vi "niRFUtil WFM Average (DVR) (complex).vi"(0 "Avg State Element DVR":T1, 5 "Data In":T2 format="%.2f", 7 "Average Mode":enum16{"Exponential", "Repeat"}(ring), 11 "error in (no error)":errorcluster, 12 "Reset?":bool=TRUE, 13 "Initialize?":bool=TRUE) -> (6 "Average Data Out":T2 format="%.2f", 8 "Average Count":i32, 15 "error out":errorcluster)   [LabVIEW 2015, in "niRFUtil.lvlib"]
doc: "(c) Copyright 2006, National Instruments, Inc. This VI may not be duplicated, sold, or distributed without written consent from National Instruments."
uses:
  niRFUtil.lvlib
  Includes/niRFUtil INC Complex Array.ctl
  Includes/niRFUtil INC Average State Reference (complex).ctl
  Includes/niRFUtil INC Average State Data (complex).ctl
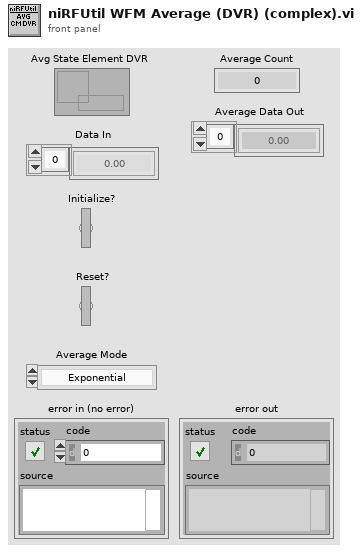
[diagram p1: front panel]
types:
  T1 = typedef "niRFUtil.lvlib/niRFUtil INC Average State Reference (complex).ctl" = refnum<data-value>
  T2 = typedef "niRFUtil.lvlib/niRFUtil INC Complex Array.ctl" = csg[]
  T3 = typedef "niRFUtil.lvlib/niRFUtil INC Average State Data (complex).ctl" = cluster{"Accumulator":T2, "Count":i32}
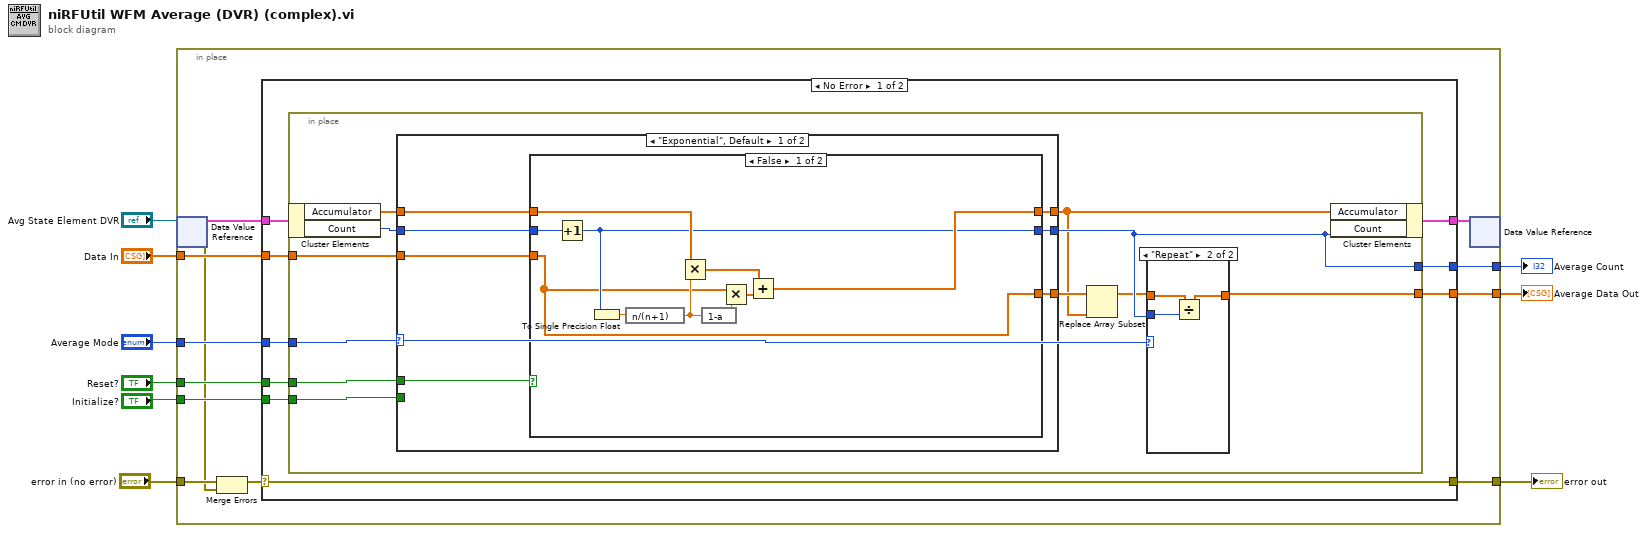
[diagram p0: block diagram]
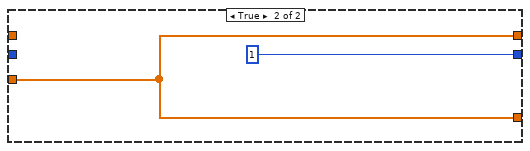
[diagram p2: hidden frame]
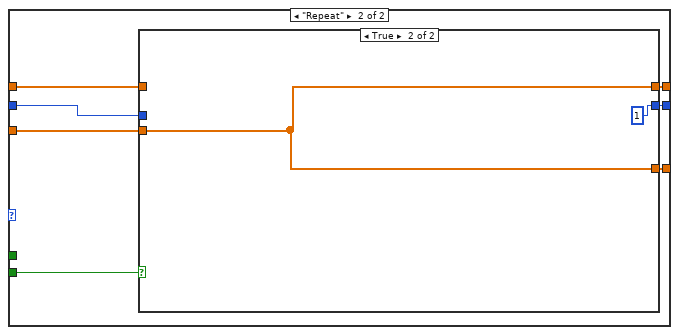
[diagram p3: hidden frame]
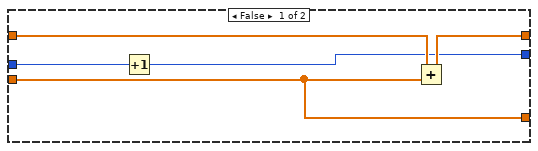
[diagram p4: hidden frame]
diagram:
  n1 = in-place {
    in-place-border: "Data In" -> [w21]
    in-place-border: "Average Mode" -> [w20]
    in-place-border: "Reset?" -> [w19]
    in-place-border: "Initialize?" -> [w18]
    in-place-border: [w17] -> w5
    in-place-border: [w14] -> w3
    in-place-border: "error in (no error)" -> [w12]
    in-place-border: [w13] -> w1
    n2 = in-place-dvr #1("Avg State Element DVR") -> (w16:T3, w11:errorcluster)
    n3 = Merge Errors(w12, w11) -> (w10:errorcluster)
    n4 = case shown="No Error" w10 {
      selector: w10 -> [w22 w79]
      tunnel: w21 -> [w30 w80]
      tunnel: w20 -> [w29 _]
      tunnel: w19 -> [w28 _]
      tunnel: w18 -> [w27 _]
      tunnel: [w26 w80] -> w17
      tunnel: w16 -> [w25 w81]
      tunnel: [w24 w81] -> w15
      tunnel: [w23 _] -> w14
      tunnel: [w22 w79] -> w13
      frame No Error {
        n5 = in-place {
          in-place-border: w30 -> [w41]
          in-place-border: w29 -> [w40]
          in-place-border: w28 -> [w39]
          in-place-border: w27 -> [w38]
          in-place-border: [w35] -> w26
          in-place-border: [w34] -> w23
          n6 = in-place-cluster #2(w25) -> ("Accumulator"=w37:T2, "Count"=w36:i32)
          n7 = case shown="\"Exponential\", Default" w40 {
            tunnel: w39 -> [w45 _]
            tunnel: [w48 w67] -> w32
            tunnel: w41 -> [w43 w62]
            tunnel: [w44 w64] -> w34
            tunnel: w37 -> [w47 w66]
            tunnel: w36 -> [w46 w65]
            tunnel: w38 -> [_ w63]
            tunnel: [w42 w61] -> w33
            frame "Exponential", Default {
              n8 = case shown="False" w45 {
                tunnel: w43 -> [w49 w59]
                tunnel: [w53 w59] -> w48
                tunnel: w47 -> [w52 _]
                tunnel: w46 -> [w51 _]
                tunnel: [w50 1] -> w44
                tunnel: [w49 w59] -> w42
                frame False {
                  n9 = Increment(x=w51) -> (x+1=w50:i32)
                  n10 = To Single Precision Float(number=w50) -> (single precision float=w58:sgl)
                  n11 = expression code="n/(n+1)"(w58) -> (w57:sgl)
                  n12 = Multiply(x=w52, y=w57) -> (x*y=w54:T2)
                  n13 = expression code="1-a"(w57) -> (w56:sgl)
                  n14 = Multiply(x=w49, y=w56) -> (x*y=w55:T2)
                  n15 = Add(x=w54, y=w55) -> (x+y=w53:T2)
                }
                frame True {
                }
              }
            }
            frame "Repeat" {
              n16 = case shown="True" w63 {
                tunnel: w62 -> [w68 w73]
                tunnel: [w72 w73] -> w67
                tunnel: w66 -> [w71 _]
                tunnel: w65 -> [w70 _]
                tunnel: [w69 1] -> w64
                tunnel: [w68 w73] -> w61
                frame False {
                  n17 = Increment(x=w70) -> (x+1=w69:i32)
                  n18 = Add(x=w71, y=w68) -> (x+y=w72:T2)
                }
                frame True {
                }
              }
            }
          }
          n19 = Replace Array Subset(array=w33, new element=w32) -> (w31:T2)  [unwired: 1 in]
          n20 = case shown="\"Repeat\"" w40 {
            tunnel: [w75 w76] -> w35
            tunnel: w31 -> [w75 w77]
            tunnel: w34 -> [_ w78]
            frame "Exponential", Default {
            }
            frame "Repeat" {
              n21 = Divide(x=w77, y=w78) -> (x/y=w76:T2)
            }
          }
          n22 = in-place-cluster #2("Accumulator"=w32, "Count"=w34) -> (w24:T3)
        }
      }
      frame Error {
      }
    }
    n23 = in-place-dvr #1(w15) -> ()  [unwired: 2 out]
  }
  "Average Data Out" <- w5
  "Average Count" <- w3
  "error out" <- w1
